vi "LoadTbl1 (SubVI).vi"(8 "error in":errorcluster, 11 "Log":refnum<vi>) -> (0 "error out":errorcluster)   [LabVIEW 2017]
uses:
  Global_SNK3_HF.vi
  LV_Unicorn/LV_Unicorn.lvlib
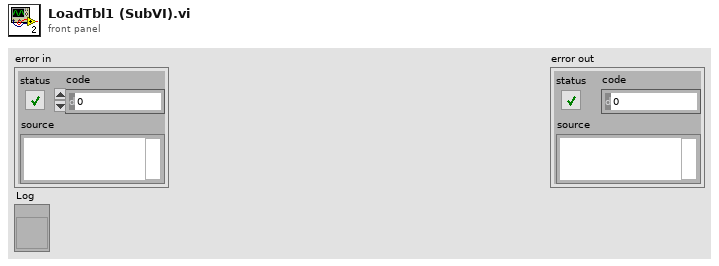
[diagram p1: front panel]
types:
  T1 = typedef "LV_Unicorn.lvlib/unicorn_Param.ctl" = cluster{"conParam":T2, "Param":T3}
  T2 = typedef "LV_Unicorn.lvlib/unicorn_conn.ctl" = cluster{"ReadIntParam":bool, "ReadDescrParam":bool, "ReadFloatParam":bool, "debug":bool, "ReadJSON":bool, "IP_address":string, "N_attempts":i32, "type_con":enum16{"Serial", "TCP"}, "MB_address":i32, "VISA":refnum<visa-resource-name>, "connection ID":refnum<k5>, "nameDevices":string, "timeout":i32, "port":u16, "type_version":string, "baud_rate":u32, "VersionControl":bool, "TCP_conn":bool, "WindowSize":i32}
  T3 = typedef "LV_Unicorn.lvlib/unicorn_JSON.ctl" = cluster{"NumParam":cluster{"NTelem":i32, "NInt":i32, "NFloat":i32, "NTable":i32}, "ParamInt":T4, "Telemetry":T5, "Table":T6, "ParamFloat":T7}
  T4 = typedef "LV_Unicorn.lvlib/unicorn_ParamInt.ctl" = cluster{"ID":string, "Num":i32, "Name":string, "Type":string, "Enum":string, "Desc":string, "Unit":string, "Access":string, "FormatStr":string, "Min":i32, "Max":i32}[]
  T5 = typedef "LV_Unicorn.lvlib/unicorn_Telemetry.ctl" = cluster{"ID":string, "Num":i32, "Name":string, "Desc":string, "Unit":string, "FormatStr":string, "Min":i32, "Max":i32}[]
  T6 = typedef "LV_Unicorn.lvlib/unicorn_Table.ctl" = cluster{"Num":i32, "Access":string, "ColumnCount":i32, "NeedParamPrepare":bool, "Columns":cluster{"Column":i32, "Desc":string, "Name":string}[], "DataType":string, "FormatStr":string, "ID":string, "Name":string, "RowCount":i32, "Rows":cluster{"Desc":string, "ID":string, "Max":i32, "Min":i32, "Name":string, "Row":i32, "Unit":string}[], "Type":string}[]
  T7 = typedef "LV_Unicorn.lvlib/unicorn_ParamFloat.ctl" = cluster{"ID":string, "Num":i32, "Name":string, "Type":string, "Enum":string, "Desc":string, "Unit":string, "Access":string, "FormatStr":string, "Min":sgl, "Max":sgl}[]
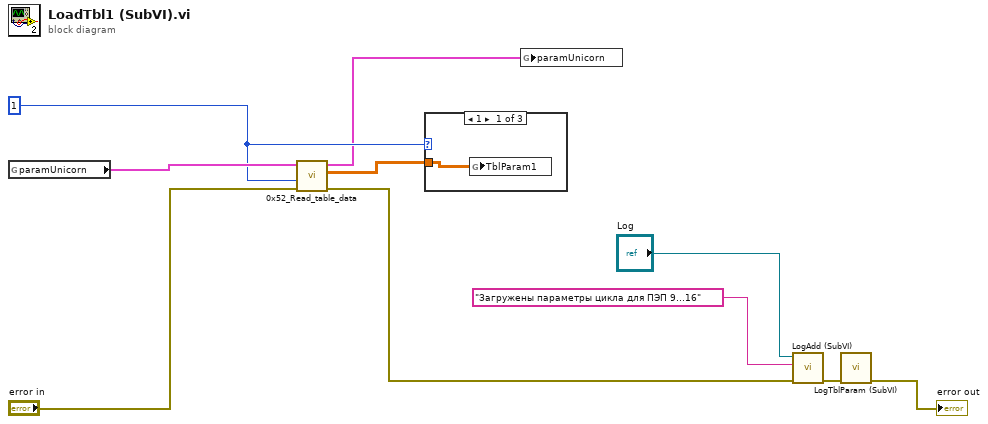
[diagram p0: block diagram]
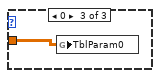
[diagram p3: hidden frame]
diagram:
  w7 = 1 ("NTable")
  n1 = global read "Global_SNK3_HF.vi" "paramUnicorn"() -> (w8:T1)
  n2 = call "0x52_Read_table_data.vi"("error in"="error in", "NTable"=w7, "paramUnicornIn"=w8) -> ("error out"=w5:errorcluster, "Array"=w4:sgl[][], "paramUnicornOut"=w3:T1)  [unwired: 6 in]
  n3 = case shown="1" w7 {
    tunnel: w4 -> [w11 _ w12]
    frame 1 {
      n4 = global write "Global_SNK3_HF.vi" "TblParam1"(w11) -> ()
    }
    frame 2, Default {
    }
    frame 0 {
      n5 = global write "Global_SNK3_HF.vi" "TblParam0"(w12) -> ()
    }
  }
  n6 = global write "Global_SNK3_HF.vi" "paramUnicorn"(w3) -> ()
  n7 = call "LogAdd (SubVI).vi"("error in"=w5, "string"="Загружены параметры цикла для ПЭП 9...16", "Log"="Log") -> ("error out"=w2:errorcluster)  [unwired: 8 in]
  n8 = call "LogTblParam (SubVI).vi"("error in"=w2) -> ("error out"=→"error out":errorcluster)  [unwired: 10 in]
